vi "ChangeSetpoint.vi"(8 "error in (no error)":errorcluster, 10 "Setpoint":dbl, 11 "SMO.TimedLoop":refnum<class "SMO.TimedLoop.lvclass">) -> (0 "error out":errorcluster, 3 "SMO.TimedLoop out":refnum<class "SMO.TimedLoop.lvclass">)   [LabVIEW 2019, in "SMO.TimedLoop.lvclass"]
doc: "---------------------------------------------------------------\nJKI State Machine Objects™\nhttp://jki.net/state-machine-objects/\nCopyright (C) 2005-2015, JKI <info@jki.net>\nALL RIGHTS RESERVEDJKI State Machine Objects (SMO) 1.0.0.5\nJKI - JKI\nCopyright (c) 2016, JKI"
uses:
  SMO.TimedLoop.lvclass
panel:
  # "For instructions on how to use the JKI State Machine Objects, examples and video tutorials, visit:\nhttp://jki.net/state-machine-objects/\n\nJKI State Machine Objects™\nhttp://jki.net/state-machine-objects/\nCopyright (C) 2005-2015, JKI <info@jki.net>\nALL RIGHTS RESERVED"
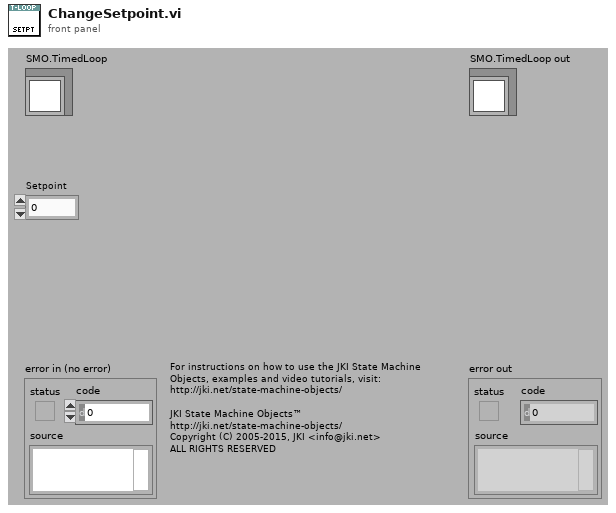
[diagram p1: front panel]
types:
  T1 = typedef "SMO.TimedLoop.lvclass/PrivateEvents--Cluster.ctl" = cluster{"AsyncMethod":refnum<user-event>}
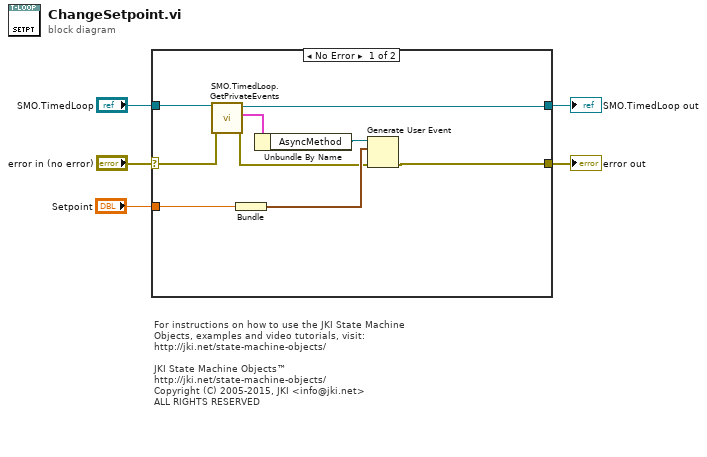
[diagram p0: block diagram]
diagram:
  # "For instructions on how to use the JKI State Machine Objects, examples and video tutorials, visit:\nhttp://jki.net/state-machine-objects/\n\nJKI State Machine Objects™\nhttp://jki.net/state-machine-objects/\nCopyright (C) 2005-2015, JKI <info@jki.net>\nALL RIGHTS RESERVED"
  n1 = case shown="No Error" "error in (no error)" {
    selector: "error in (no error)" -> [w13 w15]
    tunnel: "SMO.TimedLoop" -> [w14 w16]
    tunnel: [w6 w15] -> w4
    tunnel: [w12 w16] -> w3
    tunnel: "Setpoint" -> [w9 _]
    frame No Error {
      n2 = call "SMO.TimedLoop.GetPrivateEvents.vi"("error in (no error)"=w13, "SMO.TimedLoop"=w14) -> ("error out"=w7:errorcluster, "Private Events"=w11:T1, "SMO.TimedLoop out"=w12:refnum<class "SMO.TimedLoop.lvclass">)  [unwired: 7 in]
      n3 = Bundle("Setpoint"=w9) -> (w8:cluster{"Setpoint":dbl})  [unwired: 1 in]
      n4 = Unbundle By Name(w11) -> ("AsyncMethod"=w10:refnum<user-event>)
      n5 = Generate User Event(user event=w10, event data cluster=w8, error in=w7) -> (error out=w6:errorcluster)  [unwired: 1 in, 1 out]
    }
    frame Error {
    }
  }
  "error out" <- w4
  "SMO.TimedLoop out" <- w3
